vi "Clean Up Key String.vi"(11 "Key":string) -> (3 "Cleaned Up Key":string)   [LabVIEW 2015, in "NI_AWS_IoT.lvlib"]
uses:
  NI_AWS_IoT.lvlib
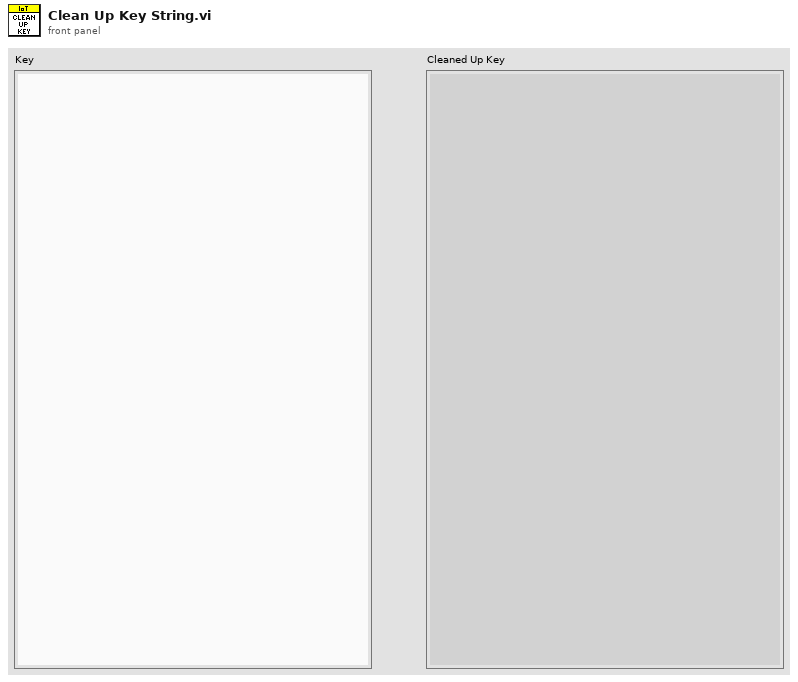
[diagram p1: front panel]
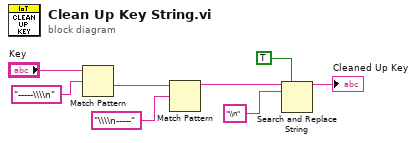
[diagram p0: block diagram]
diagram:
  n1 = Match Pattern(string="Key", regular expression="-----\\\\n") -> (after substring=w6:string)  [unwired: 1 in, 3 out]
  n2 = Match Pattern(string=w6, regular expression="\\\\n-----") -> (before substring=w4:string)  [unwired: 1 in, 3 out]
  n3 = Search and Replace String(replace all?=TRUE ("replace all? (F)"), input string=w4, search string="\\n") -> (result string=→"Cleaned Up Key":string)  [unwired: 5 in, 3 out]
